vi "mapSensorNameToId.vi"(8 "error in (no error)":errorcluster, 10 "Sensor Name":string[](array[string]), 11 "ZTAAC in":refnum<class "ZTAAC.lvclass">) -> (0 "error out":errorcluster, 2 "Sensor Id":i32[](array[numeric]), 3 "ZTAAC out":refnum<class "ZTAAC.lvclass">)   [LabVIEW 2016, in "OfcFunc.lvlib" / "ZTAAC.lvclass"]
doc: "Map the array of sensor name to sensor Id."
uses:
  ZTAAC.lvclass
  ZTAAC.lvclass/ZTAAC.ctl
  MatOper/MatOper.lvclass
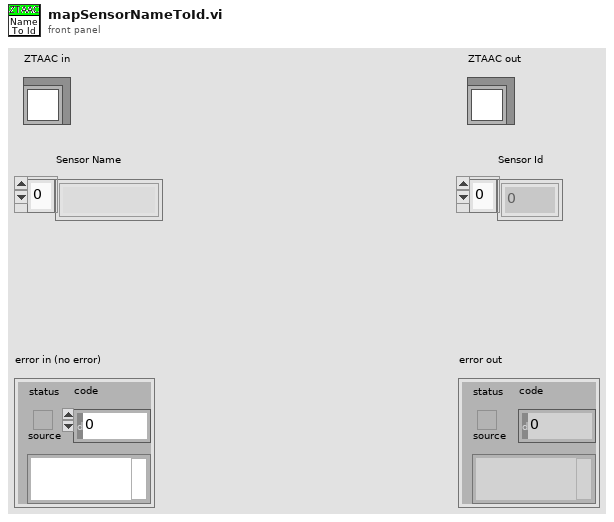
[diagram p1: front panel]
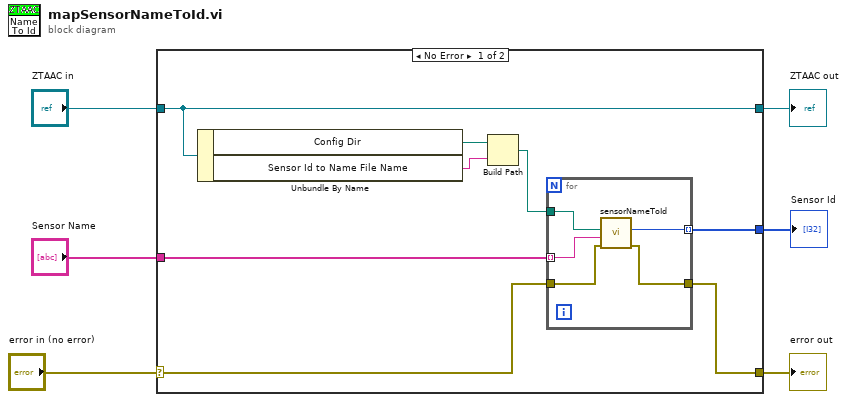
[diagram p0: block diagram]
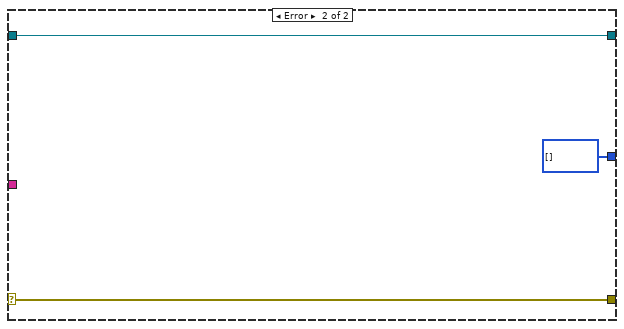
[diagram p2: hidden frame]
diagram:
  n1 = case shown="No Error" "error in (no error)" {
    selector: "error in (no error)" -> [w10 w22]
    tunnel: [w9 w22] -> w5
    tunnel: [w12 w21] -> w3
    tunnel: "ZTAAC in" -> [w12 w21]
    tunnel: "Sensor Name" -> [w8 _]
    tunnel: [w7 i32[] []] -> w1
    frame No Error {
      n2 = Unbundle By Name(w12) -> ("Config Dir"=w14:path, "Sensor Id to Name File Name"=w13:string)
      n3 = Build Path(base path=w14, name or relative path=w13) -> (appended path=w11:path)
      n4 = for {
        tunnel: w11 -> [w19]
        tunnel: w10 -> [w18]
        tunnel: [w17] -> w9
        tunnel: w8 -> [w16] mode=indexing
        tunnel: [w15] -> w7 mode=indexing
        n5 = call "sensorNameToId.vi"("error in (no error)"=w18, "Sensor Name"=w16, "Path"=w19) -> ("error out"=w17:errorcluster, "Sensor ID"=w15:i32)  [unwired: 6 in, 1 out]
      }
    }
    frame Error {
    }
  }
  "error out" <- w5
  "ZTAAC out" <- w3
  "Sensor Id" <- w1
